vi "Make Request.vi"(8 "error in (no error)":errorcluster, 11 "Session in":refnum<class "Session.lvclass">) -> (0 "error out":errorcluster, 2 "Response":T1, 3 "Session out":refnum<class "Session.lvclass">)   [LabVIEW 2015, in "NI_Azure_Core.lvlib" / "Session.lvclass"]
doc: "This core implementation of Azure HTTP requests may be used to implement special requests or API calls not present in this toolkit."
uses:
  Session.lvclass
  Response.ctl
  Signature Fields.ctl
  Name Value Pair.ctl
  Session.lvclass/Session.ctl
  Write Request body.vi
  Write HTTP Verb.vi
  Write URL Suffix.vi
  Write URL Prefix.vi
  Write Signature Fields.vi
  Write Request Parameters.vi
  Write Request Headers.vi
  Write _StorageAccountSuffix.vi
  Write _ServiceName.vi
  NI_Azure_Core.lvlib
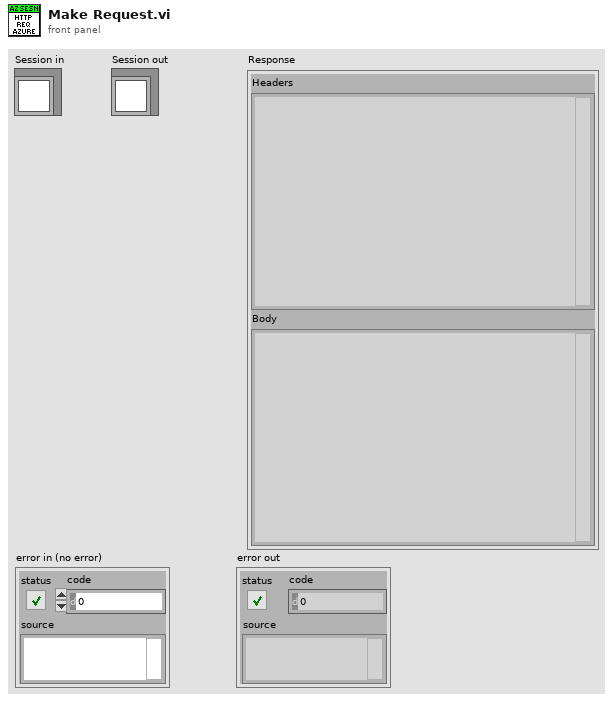
[diagram p1: front panel]
types:
  T1 = typedef "NI_Azure_Core.lvlib/Response.ctl" = cluster{"Headers":string, "Body":string}
  T2 = typedef "NI_Azure_Core.lvlib/Name Value Pair.ctl" = cluster{"name":string, "value":string}
  T3 = typedef "NI_Azure_Core.lvlib/Signature Fields.ctl" = cluster{"Content-Encoding":string, "Content-Language":string, "Content-Length":string, "Content-MD5":string, "Content-Type":string, "Date":string, "If-Modified-Since":string, "If-Match":string, "If-None-Match":string, "If-Unmodified-Since":string, "Range":string}
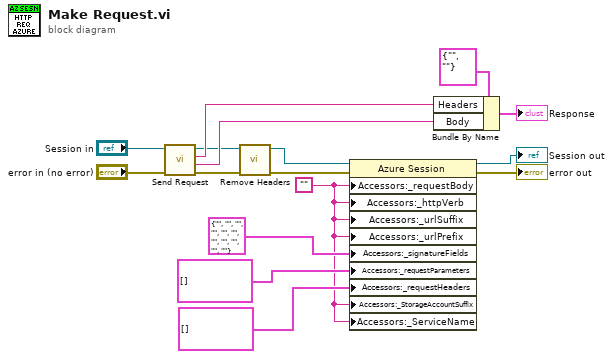
[diagram p0: block diagram]
diagram:
  w1 = "" ("_requestBody")
  n1 = call "Send Request.vi"("error in (no error)"="error in (no error)", "HTTP Session in"="Session in") -> ("error out"=w12:errorcluster, "Response body"=w11:string, "Response headers"=w10:string, "HTTP Session out"=w9:refnum<class "Session.lvclass">)  [unwired: 6 in]
  n2 = call "Remove Headers.vi"("error in (no error)"=w12, "HTTP Session in"=w9) -> ("error out"=w13:errorcluster, "HTTP Session out"=w7:refnum<class "Session.lvclass">)  [unwired: 8 in]
  n3 = property class="Azure Session"(reference=w7, error in=w13, "Accessors:_requestBody"=w1, "Accessors:_httpVerb"=w1, "Accessors:_urlSuffix"=w1, "Accessors:_urlPrefix"=w1, "Accessors:_signatureFields"=T3 {"Content-Encoding"="", "Content-Language"="", "Content-Length"="", "Content-MD5"="", "Content-Type"="", "Date"="", "If-Modified-Since"="", "If-Match"="", "If-None-Match"="", "If-Unmodified-Since"="", "Range"=""} ("_signatureFields"), "Accessors:_requestParameters"=T2[] [] ("_requestParameters"), "Accessors:_requestHeaders"=T2[] [] ("_requestHeaders"), "Accessors:_StorageAccountSuffix"=w1, "Accessors:_ServiceName"=w1) -> (reference out=→"Session out":refnum<class "Session.lvclass">, error out=→"error out":errorcluster)
  n4 = Bundle By Name(cluster=T1 {"Headers"="", "Body"=""} ("Response"), "Headers"=w10, "Body"=w11) -> (→"Response":T1)
